vi "Factory.vi"(0 "Base in":refnum<class "KDemoBase.lvclass">, 7 "Variant":variant, 9 "Prefix":string, 11 "error in (no error)":errorcluster) -> (4 "Base out":refnum<class "KDemoBase.lvclass">, 8 "Type":string, 15 "error out":errorcluster)   [LabVIEW 2015, in "KDemoBase.lvclass"]
uses:
  KDemoBase.lvclass
  KDemoDerived Class/KDemoDerived.lvclass
  KObject Class/KObject.lvclass
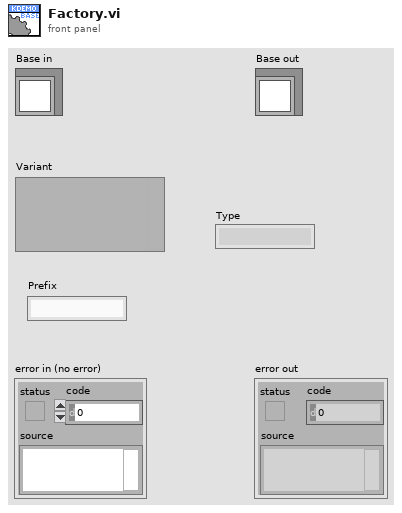
[diagram p1: front panel]
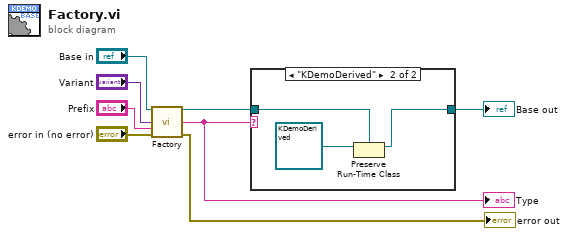
[diagram p0: block diagram]
diagram:
  n1 = call-parent "Factory.vi"("KObject in"="Base in", "Variant"="Variant", "Prefix"="Prefix", "error in (no error)"="error in (no error)") -> ("KObject out"=w2:refnum<class "KDemoBase.lvclass">, "Type"=w3:string, "error out"=→"error out":errorcluster)  [unwired: 9 in]
  "Type" <- w3
  n2 = case shown="\"KDemoDerived\"" w3 {
    tunnel: w2 -> [w9 w12]
    tunnel: [w9 w11] -> w1
    frame "0", Default {
    }
    frame "KDemoDerived" {
      n3 = Preserve Run-Time Class(object in=refnum<class "KDemoDerived.lvclass"> refnum ("Gen2"), 2:w12) -> (object out=w11:refnum<class "KDemoBase.lvclass">)  [unwired: 1 in, 1 out]
    }
  }
  "Base out" <- w1
